vi "Stimulate This.vi"(5 "Stim Channel":T2) -> (1 "Stim Status Channel":T3, 2 "Stim Log Channel":T1)   [LabVIEW 2019]
uses:
  Lee Lab/CP FES Walking 2018/Code/Working/LabVIEW/Controls/States/Stim State.ctl
  <extravilib>/ChannelInstances/Messenger-t'Stim Status Message.ctl'/))Channel.ctl
  Lee Lab/CP FES Walking 2018/Code/Working/LabVIEW/Controls/Messages/Stim Status Message.ctl
  Lee Lab/CP FES Walking 2018/Code/Working/LabVIEW/RehaStim API/Reusable Stim Module/Stimulator Status State.ctl
  <extravilib>/ChannelInstances/Messenger-t'Stim Message.ctl'/))Channel.ctl
  Lee Lab/CP FES Walking 2018/Code/Working/LabVIEW/Controls/Messages/Stim Message.ctl
  <extravilib>/ChannelInstances/Messenger-t'Log Message.ctl'/))Channel.ctl
  Lee Lab/CP FES Walking 2018/Code/Working/LabVIEW/Controls/Messages/Log Message.ctl
  Lee Lab/CP FES Walking 2018/Code/Working/LabVIEW/Controls/States/Log State.ctl
  Controls/Stim Status Cluster.ctl
  Controls/Stimulator Mode.ctl
  Controls/Stimulator Cluster.ctl
  Version 2/Data Type Defs/Pulse Mode (array).ctl
  Controls/Stim Current Array.ctl
  Controls/Pulse Duration Array.ctl
  <extravilib>/ChannelInstances/Messenger-t'Stim Message.ctl'/Read With Abort.vi
  <extravilib>/ChannelInstances/Messenger-t'Stim Message.ctl'/Write With Abort.vi
  <extravilib>/ChannelInstances/Messenger-t'Log Message.ctl'/Write With Abort.vi
  <extravilib>/ChannelInstances/Messenger-t'Stim Status Message.ctl'/Write With Abort.vi
  <resource>/Channels/Messenger/Read With Abort.vi
  <vilib>/ChannelSupport/Channel Message/Read ID.vi
  <resource>/Channels/Messenger/Write With Abort.vi
  <extravilib>/ChannelInstances/Messenger-t'Stim Message.ctl'/Wrapper.lvclass
  C:/Program Files/National Instruments/LabVIEW 2019/vi.lib/ChannelSupport/Channel Message/Channel Message.lvclass
  <extravilib>/ChannelInstances/Messenger-t'Log Message.ctl'/Wrapper.lvclass
  <extravilib>/ChannelInstances/Messenger-t'Stim Status Message.ctl'/Wrapper.lvclass
  <resource>/Channels/Messenger/Endpoint.vi
  <extravilib>/ChannelInstances/Messenger-t'Stim Message.ctl'/Unwrap.vi
  <extravilib>/ChannelInstances/Messenger-t'Stim Message.ctl'/Wrap.vi
  <extravilib>/ChannelInstances/Messenger-t'Log Message.ctl'/Wrap.vi
  <extravilib>/ChannelInstances/Messenger-t'Stim Status Message.ctl'/Wrap.vi
  <extravilib>/ChannelInstances/Messenger-t'Stim Message.ctl'.lvlib
  <extravilib>/ChannelInstances/Messenger-t'Log Message.ctl'.lvlib
  <extravilib>/ChannelInstances/Messenger-t'Stim Status Message.ctl'.lvlib
panel:
  out "Stim State":T4=enum."Idle"
  out "Stim":i32
  out "Stim On/Off":bool
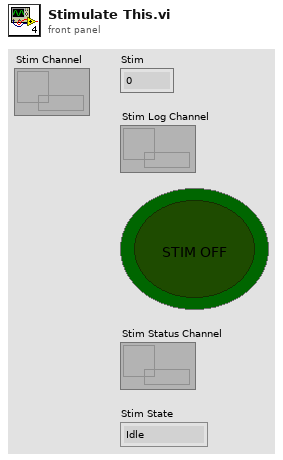
[diagram p1: front panel]
types:
  T1 = typedef "Messenger-t'Log Message.ctl'.lvlib/))Channel.ctl" = refnum<queue>
  T2 = typedef "Messenger-t'Stim Message.ctl'.lvlib/))Channel.ctl" = refnum<queue>
  T3 = typedef "Messenger-t'Stim Status Message.ctl'.lvlib/))Channel.ctl" = refnum<queue>
  T4 = typedef "Stim State.ctl" = enum16{"Initialize", "Open", "Idle", "Start Stim", "Update Params", "GPD Update", "Stop Stim", "Close", "Quit", "Clear Log"}
  T5 = typedef "Stim Message.ctl" = cluster{"Stim State":T4, "Data":variant}
  T6 = typedef "Stimulator Mode.ctl" = string
  T7 = cluster{"Name":refnum<visa-resource-name>, "Open":bool, " Mode":T6}
  T8 = typedef "Stim Status Message.ctl" = cluster{"Stimulator State":T9, "Data":variant}
  T9 = typedef "Stimulator Status State.ctl" = enum16{"Update"}
  T10 = typedef "Stim Status Cluster.ctl" = cluster{"Stim On/Off":bool, "Stim State":T4}
  T11 = cluster{"Doublet/Triplet Interval":dbl, "N factor":u8, "Stim Frequency":dbl, "Active Channels":bool[], "Low-Frequency Channels":bool[]}
  T12 = typedef "Stimulator Cluster.ctl" = cluster{"Log File In":refnum<file>, "Stimulator In":refnum<visa-resource-name>, "Stimulator Mode":T6, "Log Data":bool, "Doublet/Triplet  Interval":dbl, "Stim Frequency":dbl, "N-Factor":u8, "Active Channels":bool[], "Low-Frequency Channels":bool[], "Stimulator State":enum16{"Closed", "Open", "Initialized", "Stimulating"}, "Mode Array":T13, "Current Array":T14, "Pulse Duration Array":T15, "VISA Timeout":u32}
  T13 = typedef "Pulse Mode (array).ctl" = enum16{"Single", "Doublet", "Triplet"}[]
  T14 = typedef "Stim Current Array.ctl" = u8[]
  T15 = typedef "Pulse Duration Array.ctl" = u32[]
  T16 = typedef "Log Message.ctl" = cluster{"Log State":T17, "Data":variant}
  T17 = typedef "Log State.ctl" = enum16{"Open", "Initialize", "Update", "On", "Off", "Idle", "Close", "Quit"}
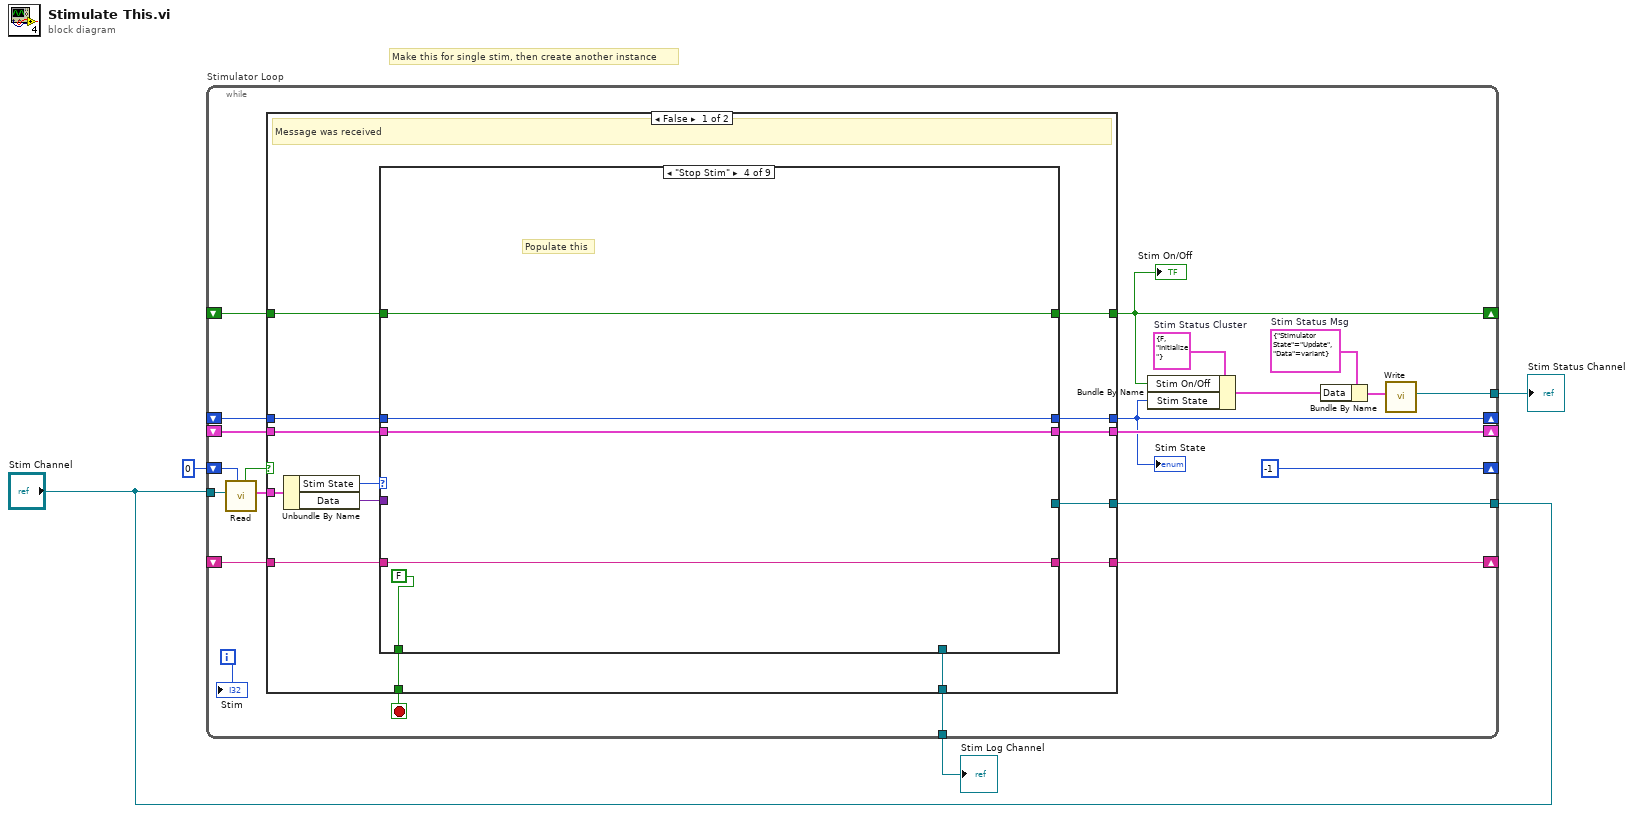
[diagram p0: block diagram]
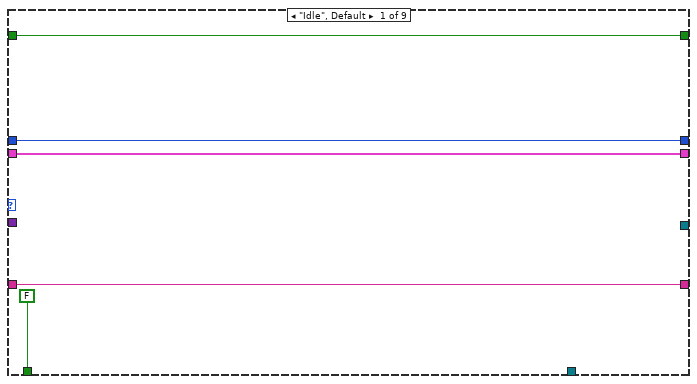
[diagram p2: hidden frame]
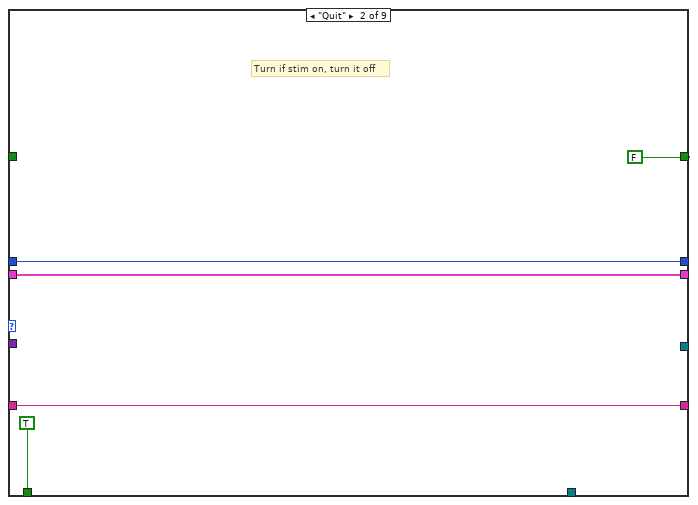
[diagram p3: hidden frame]
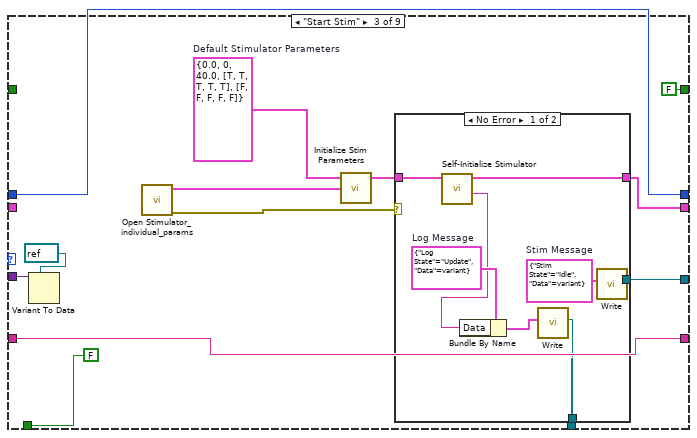
[diagram p4: hidden frame]
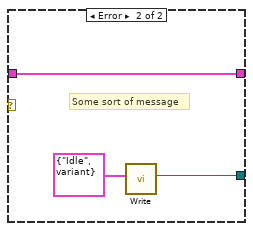
[diagram p5: hidden frame]
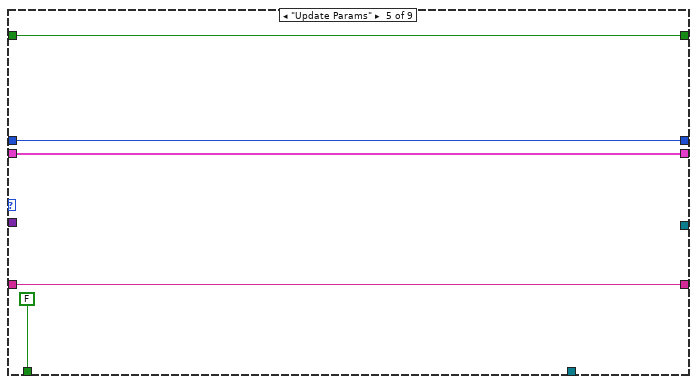
[diagram p6: hidden frame]
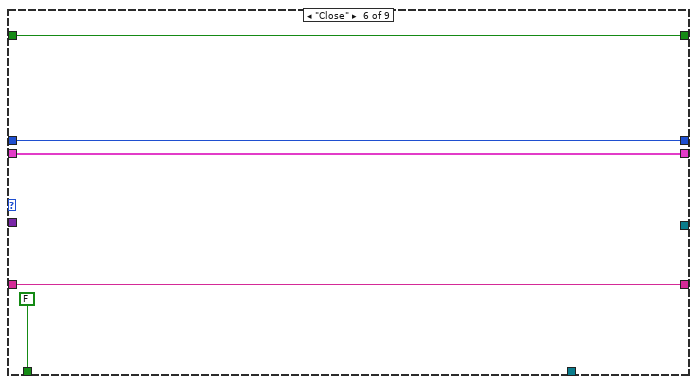
[diagram p7: hidden frame]
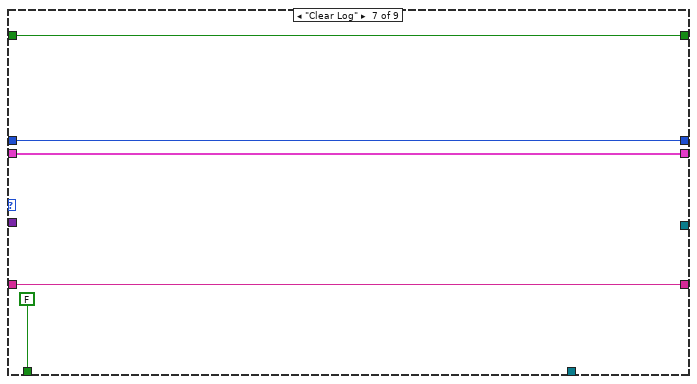
[diagram p8: hidden frame]
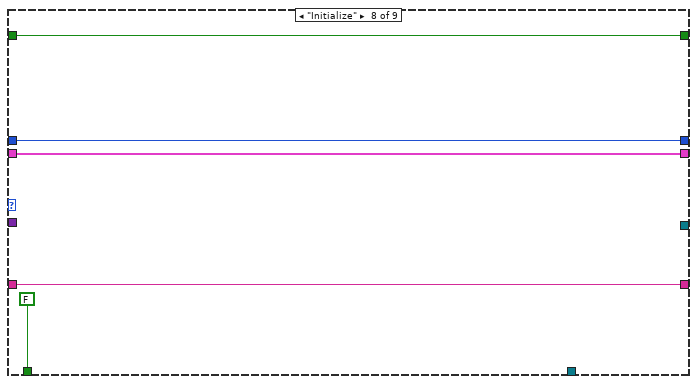
[diagram p9: hidden frame]
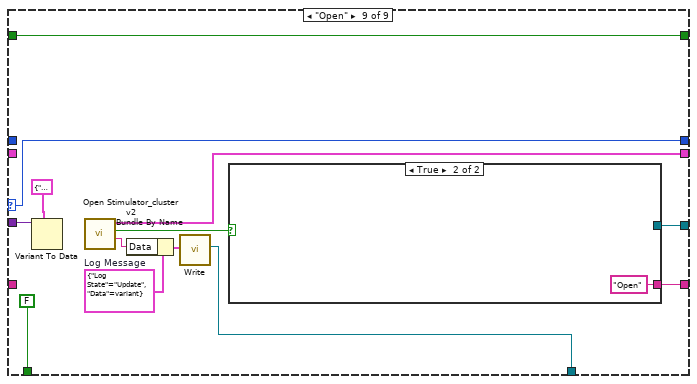
[diagram p10: hidden frame]
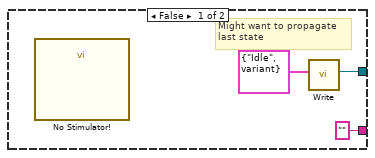
[diagram p11: hidden frame]
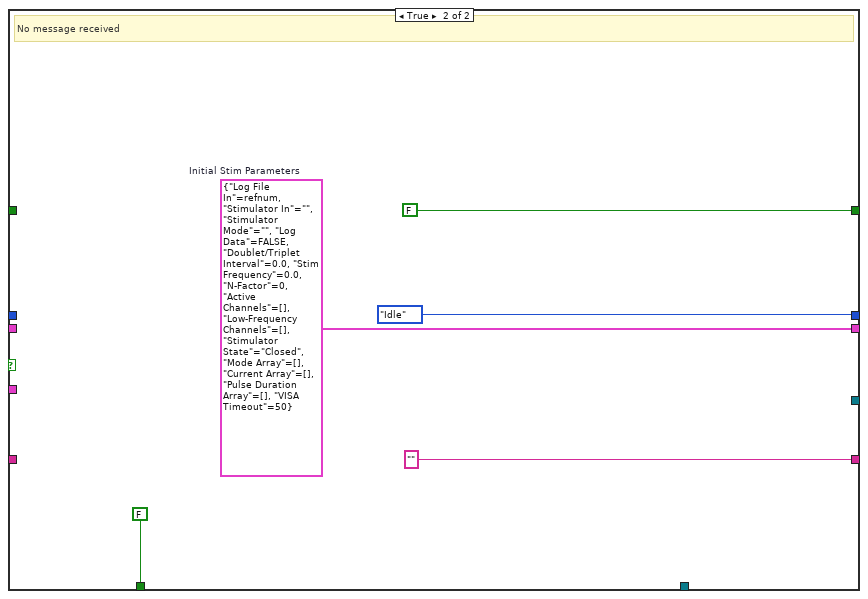
[diagram p12: hidden frame]
diagram:
  # "Make this for single stim, then create another instance"
  n1 = while "Stimulator Loop" {
    tunnel: "Stim Channel" -> [w23]
    shift-right: [w26] -> _
    shift-left: _ -> [w25]
    tunnel: "Stim Channel" -> [w22]
    shift-right: [w11] -> _
    shift-left: _ -> [w18]
    shift-right: [w10] -> _
    shift-left: _ -> [w17]
    shift-right: [w16] -> _
    shift-left: _ -> [w15]
    tunnel: [w14] -> w1
    shift-right: [-1] -> _
    shift-left: 0 -> [w13]
    tunnel: [w5] -> w4
    i -> [w21]
    stop <- w24 stop-if-true
    w8 = T8 {"Stimulator State"=enum."Update", "Data"=variant}  # Stim Status Msg
    w9 = T10 {"Stim On/Off"=FALSE, "Stim State"=enum."Initialize"}  # Stim Status Cluster
    n2 = call <extravilib>:"Read.vi"("timeout in ms (-1)"=w13, "channel"=w23) -> ("element"=w20:T5, "timedout?"=w19:bool)  [unwired: 6 in, 2 out]
    n3 = case shown="False" w19 {
      tunnel: [w40 w119] -> w26
      tunnel: w25 -> [w39 _]
      tunnel: [w38 FALSE] -> w24
      tunnel: [w37 _] -> w22
      tunnel: [w36 FALSE ("Stim On/Off")] -> w11
      tunnel: w20 -> [w35 _]
      tunnel: w18 -> [w32 _]
      tunnel: w17 -> [w31 _]
      tunnel: [w30 Stim_State."Idle" ("Stim State")] -> w10
      tunnel: [w29 "" ("Stim State")] -> w16
      tunnel: w15 -> [w28 _]
      tunnel: [w27 _] -> w14
      frame False {
        # "Message was received"
        n4 = Unbundle By Name(w35) -> ("Stim State"=w34:T4, "Data"=w33:variant)
        n5 = case shown="\"Stop Stim\"" w34 {
          selector: w34 -> [_ _ _ _ _ _ _ _ w111]
          tunnel: w33 -> [_ _ w57 _ _ _ _ _ w112]
          tunnel: [w45 w50 w61 w79 w82 w87 w92 w97 w110] -> w40
          tunnel: [_ _ w60 _ _ _ _ _ w104] -> w37
          tunnel: w39 -> [w45 w50 _ w79 w82 w87 w92 w97 _]
          tunnel: [FALSE TRUE FALSE FALSE FALSE FALSE FALSE FALSE FALSE] -> w38
          tunnel: [w43 FALSE ("Stim On/Off") FALSE ("Stim On/Off") w77 w84 w89 w94 w99 w100] -> w36
          tunnel: w32 -> [w43 _ _ w77 w84 w89 w94 w99 w100]
          tunnel: w31 -> [w42 w46 w53 w76 w83 w88 w93 w98 _]
          tunnel: [w42 w46 w53 w76 w83 w88 w93 w98 w111] -> w30
          tunnel: [w41 w47 w54 w75 w81 w86 w91 w96 w103] -> w29
          tunnel: w28 -> [w41 w47 w54 w75 w81 w86 w91 w96 _]
          tunnel: [_ _ w51 _ _ _ _ _ w101] -> w27
          frame "Idle", Default {
          }
          frame "Quit" {
            # "Turn if stim on, turn it off"
          }
          frame "Start Stim" {
            w62 = T11 {"Doublet/Triplet Interval"=0.0, "N factor"=0, "Stim Frequency"=40.0, "Active Channels"=[TRUE, TRUE, TRUE, TRUE, TRUE], "Low-Frequency Channels"=[FALSE, FALSE, FALSE, FALSE, FALSE]}  # Default Stimulator Parameters
            n6 = Variant To Data(type=refnum<visa-resource-name> refnum ("Left Stimulator"), Variant=w57) -> ()  [unwired: 1 in, 2 out]
            n7 = call "Open Stimulator_individual_params.vi"() -> ("error IO"=w52:errorcluster, "Stimulator"=w56:T12)  [unwired: 4 in, 2 out]
            n8 = call "Initialize Stim Parameters.vi"("Stimulator in"=w56, "Default Stimulator Parameters"=w62) -> ("Stimulator out"=w63:T12)  [unwired: 3 in]
            n9 = case shown="No Error" w52 {
              tunnel: w63 -> [w71 w74]
              tunnel: [w70 w74] -> w61
              tunnel: [w68 w72] -> w60
              tunnel: [w64 _] -> w51
              frame No Error {
                w67 = T16 {"Log State"=enum."Update", "Data"=variant}  # Log Message
                w69 = T5 {"Stim State"=enum."Idle", "Data"=variant}  # Stim Message
                n10 = call "Self-Initialize Stimulator.vi"("Stimulator in"=w71) -> ("Write to Log"=w66:string, "Stimulator Out"=w70:T12)  [unwired: 3 in, 2 out]
                n11 = Bundle By Name(cluster=w67, "Data"=w66) -> (w65:T16)
                n12 = call <extravilib>:"Write.vi"("element"=w65) -> ("channel"=w64:T1)  [unwired: 8 in, 2 out]
                n13 = call <extravilib>:"Write.vi"("element"=w69) -> ("channel"=w68:T2)  [unwired: 8 in, 2 out]
              }
              frame Error {
                # "Some sort of message"
                n14 = call <extravilib>:"Write.vi"("element"=T5 {"Stim State"=enum."Idle", "Data"=variant}) -> ("channel"=w72:T2)  [unwired: 8 in, 2 out]
              }
            }
          }
          frame "Stop Stim" {
            # "Populate this"
          }
          frame "Update Params" {
          }
          frame "Close" {
          }
          frame "Clear Log" {
          }
          frame "Initialize" {
          }
          frame "Open" {
            w109 = T16 {"Log State"=enum."Update", "Data"=variant}  # Log Message
            n15 = Variant To Data(type=T7 {"Name"="", "Open"=FALSE, " Mode"=""} ("Left Stimulator Control"), Variant=w112) -> ()  [unwired: 1 in, 2 out]
            n16 = call "Open Stimulator_cluster v2.vi"() -> ("Log Entry"=w108:string, "Stim Open"=w106:bool, "Stimulator"=w110:T12)  [unwired: 5 in]
            n17 = Bundle By Name(cluster=w109, "Data"=w108) -> (w107:T16)
            n18 = call <extravilib>:"Write.vi"("element"=w107) -> ("channel"=w101:T1)  [unwired: 8 in, 2 out]
            n19 = case shown="True" w106 {
              tunnel: [w114 _] -> w104
              tunnel: ["" ("Stim State") "Open" ("Stim State")] -> w103
              frame False {
                # "Might want to propagate\nlast state"
                n20 = call "No Stimulator!"() -> ()  [unwired: 18 in, 2 out]
                n21 = call <extravilib>:"Write.vi"("element"=T5 {"Stim State"=enum."Idle", "Data"=variant}) -> ("channel"=w114:T2)  [unwired: 8 in, 2 out]
              }
              frame True {
              }
            }
          }
        }
      }
      frame True {
        w119 = T12 {"Log File In"=refnum, "Stimulator In"="", "Stimulator Mode"="", "Log Data"=FALSE, "Doublet/Triplet  Interval"=0.0, "Stim Frequency"=0.0, "N-Factor"=0, "Active Channels"=[], "Low-Frequency Channels"=[], "Stimulator State"=enum."Closed", "Mode Array"=[], "Current Array"=[], "Pulse Duration Array"=[], "VISA Timeout"=50}  # Initial Stim Parameters
        # "No message received"
      }
    }
    "Stim On/Off" <- w11
    "Stim State" <- w10
    n22 = Bundle By Name(cluster=w9, "Stim On/Off"=w11, "Stim State"=w10) -> (w7:T10)
    n23 = Bundle By Name(cluster=w8, "Data"=w7) -> (w6:T8)
    n24 = call <extravilib>:"Write.vi"("element"=w6) -> ("channel"=w5:T3)  [unwired: 8 in, 2 out]
    "Stim" <- w21
  }
  "Stim Status Channel" <- w4
  "Stim Log Channel" <- w1
